vi "Weibull Inverse CDF.vi"(9 "b":dbl=3.0, 10 "a":dbl=1.0, 11 "cdf(x)":dbl=0.6321205588285577) -> (0 "error":i32, 3 "x":dbl=1.0000000060900718)   [LabVIEW 2017, in "NI_Gmath.lvlib"]
doc: "Computes the continuous inverse cumulative distribution function (CDF) of the various distributions. You must manually select the polymorphic instance to use."
uses:
  NI_Gmath.lvlib
  st_error_code.ctl
panel:
  # "Weibull Inverse CDF"
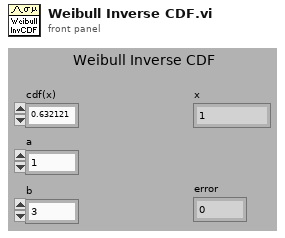
[diagram p1: front panel]
types:
  T1 = typedef "NI_Gmath.lvlib/st_error_code.ctl" = i32
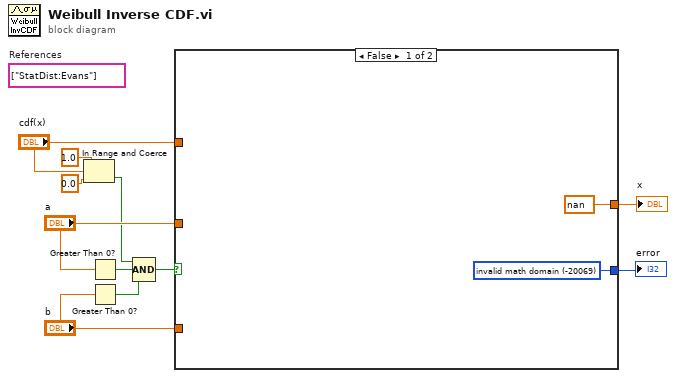
[diagram p0: block diagram]
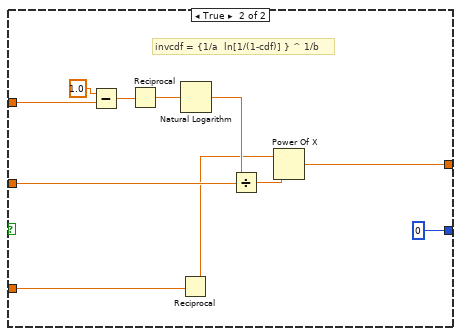
[diagram p2: hidden frame]
diagram:
  (unwired) string[] ["StatDist:Evans"]  # References
  n1 = In Range and Coerce(upper limit=1.0, x="cdf(x)", lower limit=0.0) -> (In Range?=w1:bool)  [unwired: 1 out]
  n2 = Greater Than 0?(x="a") -> (x > 0?=w2:bool)
  n3 = Greater Than 0?(x="b") -> (x > 0?=w3:bool)
  n4 = Compound Arithmetic op=AND(w1, w2, w3) -> (w4:bool)
  n5 = case shown="False" w4 {
    tunnel: "b" -> [_ w19]
    tunnel: [w12 0 ("invalid math domain")] -> w11
    tunnel: [nan w14] -> w10
    tunnel: "cdf(x)" -> [_ w22]
    tunnel: "a" -> [_ w18]
    frame False {
      w12 = T1 -20069 items=["invalid math domain"=-20069, "Fourier interpolation size m >= n"=-20070, "empty array"=-20003] ("stat interp error code")
    }
    frame True {
      # "invcdf = {1/a  ln[1/(1-cdf)] } ^ 1/b"
      n6 = Subtract(x=1.0, y=w22) -> (x-y=w21:dbl)
      n7 = Reciprocal(x=w21) -> (1/x=w20:dbl)
      n8 = Reciprocal(x=w19) -> (1/x=w15:dbl)
      n9 = Natural Logarithm(1:w20) -> (0:w17:dbl)
      n10 = Divide(x=w17, y=w18) -> (x/y=w16:dbl)
      n11 = Power Of X(1:w16, 2:w15) -> (0:w14:dbl)
    }
  }
  "x" <- w10
  "error" <- w11
